vi "LogSettings.vi"(6 "ScriptName":string, 7 "Operation":T2, 8 "error in (no error)":errorcluster, 11 "Log Settings":T1) -> (0 "error out":errorcluster, 3 "Settings out":T1)   [LabVIEW 2011]
uses:
  Strict Type Controls/Settings Operation.ctl
  <vilib>/Utility/config.llb/Read Key (String).vi
  <vilib>/Utility/config.llb/Write Key (String).vi
  <vilib>/Utility/config.llb/NI_LVConfig.lvlib
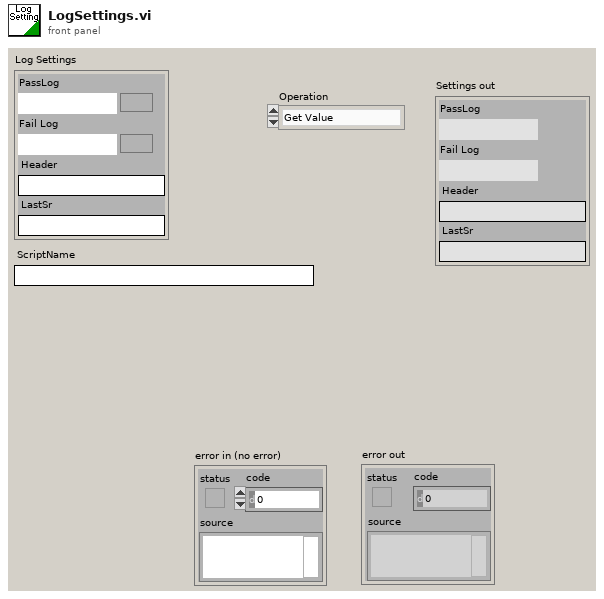
[diagram p1: front panel]
types:
  T1 = cluster{"PassLog":path, "Fail Log":path, "Header":string, "LastSr":string}
  T2 = typedef "Settings Operation.ctl" = enum8{"Get Value", "Set Value", "Read File", "Write File", "Write Stored Value"}
  T3 = typedef "NI_LVConfig.lvlib/Config Data RefNum.ctl" = refnum<k1>
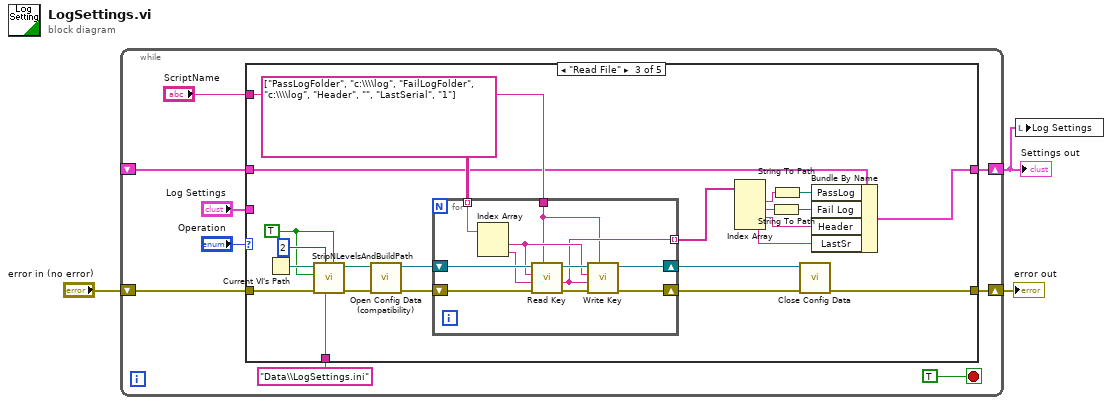
[diagram p0: block diagram]
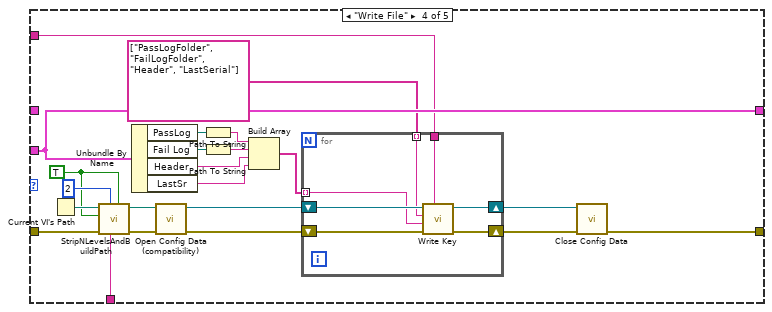
[diagram p4: hidden frame]
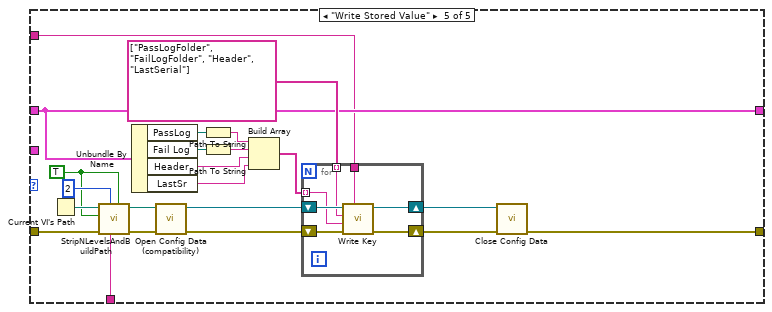
[diagram p5: hidden frame]
diagram:
  n1 = while {
    shift-right: [w11] -> w1
    shift-left: _ -> [w12]
    shift-right: [w8] -> w2
    shift-left: "error in (no error)" -> [w9]
    stop <- TRUE stop-if-true
    n2 = case shown="\"Read File\"" "Operation" {
      tunnel: w12 -> [w14 _ w27 _ w82]
      tunnel: [w14 w16 w26 w62 w82] -> w11
      tunnel: "Log Settings" -> [_ w16 _ w62 _]
      tunnel: w9 -> [w13 w15 w34 w71 w100]
      tunnel: [w13 w15 w18 w66 w95] -> w8
      tunnel: "Data\\LogSettings.ini" ("Build Path") -> [_ _ w33 w65 w94]
      tunnel: "ScriptName" -> [_ _ w28 w52 w81]
      frame "Get Value" {
      }
      frame "Set Value" {
      }
      frame "Read File" {
        w37 = TRUE ("Is File?")
        n3 = Current VI's Path() -> (path=w39:path)
        n4 = call "StripNLevelsAndBuildPath.vi"("Create Folders"=w37, "Build Path"=w33, "Strip Levels"=2, "error in(no error)"=w34, "Is File"=w37, "Path In"=w39) -> ("error out"=w35:errorcluster, "Path Out"=w36:path)  [unwired: 4 out]
        n5 = call <vilib>:"Open Config Data (compatibility).vi"("error in (no error)"=w35, "configuration file path"=w36) -> ("error out"=w32:errorcluster, "refnum"=w31:T3)  [unwired: 7 in, 1 out]
        n6 = for {
          shift-right: [w43] -> w30
          shift-left: w31 -> [w50]
          shift-right: [w45] -> w19
          shift-left: w32 -> [w49]
          tunnel: string[][] [["PassLogFolder", "c:\\\\log"], ["FailLogFolder", "c:\\\\log"], ["Header", ""], ["LastSerial", "1"]] ("appended array") -> [w48] mode=indexing
          tunnel: w28 -> [w40]
          tunnel: [w41] -> w25 mode=indexing
          n7 = Index Array(array=w48) -> (element #1=w42:string, element #2=w47:string)  [unwired: 2 in]
          n8 = call-poly <vilib>:"Read Key.vi"("section"=w40, "error in (no error)"=w49, "default value"=w47, "key"=w42, "refnum"=w50) -> ("error out"=w46:errorcluster, "value"=w41:string, "refnum out"=w44:T3)  [unwired: 1 in, 3 out]
          n9 = call-poly <vilib>:"Write Key.vi"("section"=w40, "error in (no error)"=w46, "value"=w41, "key"=w42, "refnum"=w44) -> ("error out"=w45:errorcluster, "refnum out"=w43:T3)  [unwired: 1 in, 4 out]
        }
        n10 = Index Array(array=w25) -> (element #1=w22:string, element #2=w24:string, element #3=w20:string, element #4=w17:string)  [unwired: 4 in]
        n11 = String To Path(string=w24) -> (path=w23:path)
        n12 = String To Path(string=w22) -> (path=w21:path)
        n13 = call <vilib>:"Close Config Data.vi"("error in (no error)"=w19, "refnum"=w30) -> ("error out"=w18:errorcluster)  [unwired: 1 in, 8 out]
        n14 = Bundle By Name(cluster=w27, "PassLog"=w21, "Fail Log"=w23, "Header"=w20, "LastSr"=w17) -> (w26:T1)
      }
      frame "Write File" {
        w69 = TRUE ("Is File?")
        n15 = Current VI's Path() -> (path=w72:path)
        n16 = call "StripNLevelsAndBuildPath.vi"("Create Folders"=w69, "Build Path"=w65, "Strip Levels"=2, "error in(no error)"=w71, "Is File"=w69, "Path In"=w72) -> ("error out"=w67:errorcluster, "Path Out"=w68:path)  [unwired: 4 out]
        n17 = Unbundle By Name(w62) -> ("PassLog"=w60:path, "Fail Log"=w61:path, "Header"=w55:string, "LastSr"=w51:string)
        n18 = call <vilib>:"Open Config Data (compatibility).vi"("error in (no error)"=w67, "configuration file path"=w68) -> ("error out"=w63:errorcluster, "refnum"=w64:T3)  [unwired: 7 in, 1 out]
        n19 = Path To String(path=w60) -> (string=w56:string)
        n20 = Path To String(path=w61) -> (string=w57:string)
        n21 = Build Array(w56, w57, w55, w51) -> (w54:string[])
        n22 = for {
          tunnel: w54 -> [w75] mode=indexing
          shift-right: [w77] -> w59
          shift-left: w64 -> [w79]
          shift-right: [w76] -> w58
          shift-left: w63 -> [w78]
          tunnel: string[] ["PassLogFolder", "FailLogFolder", "Header", "LastSerial"] ("appended array") -> [w74] mode=indexing
          tunnel: w52 -> [w73]
          n23 = call-poly <vilib>:"Write Key.vi"("section"=w73, "error in (no error)"=w78, "value"=w75, "key"=w74, "refnum"=w79) -> ("error out"=w76:errorcluster, "refnum out"=w77:T3)  [unwired: 1 in, 4 out]
        }
        n24 = call <vilib>:"Close Config Data.vi"("error in (no error)"=w58, "refnum"=w59) -> ("error out"=w66:errorcluster)  [unwired: 1 in, 8 out]
      }
      frame "Write Stored Value" {
        w98 = TRUE ("Is File?")
        n25 = Current VI's Path() -> (path=w101:path)
        n26 = call "StripNLevelsAndBuildPath.vi"("Create Folders"=w98, "Build Path"=w94, "Strip Levels"=2, "error in(no error)"=w100, "Is File"=w98, "Path In"=w101) -> ("error out"=w96:errorcluster, "Path Out"=w97:path)  [unwired: 4 out]
        n27 = Unbundle By Name(w82) -> ("PassLog"=w90:path, "Fail Log"=w91:path, "Header"=w85:string, "LastSr"=w80:string)
        n28 = call <vilib>:"Open Config Data (compatibility).vi"("error in (no error)"=w96, "configuration file path"=w97) -> ("error out"=w92:errorcluster, "refnum"=w93:T3)  [unwired: 7 in, 1 out]
        n29 = Path To String(path=w90) -> (string=w86:string)
        n30 = Path To String(path=w91) -> (string=w87:string)
        n31 = Build Array(w86, w87, w85, w80) -> (w84:string[])
        n32 = for {
          tunnel: w84 -> [w104] mode=indexing
          shift-right: [w106] -> w89
          shift-left: w93 -> [w108]
          shift-right: [w105] -> w88
          shift-left: w92 -> [w107]
          tunnel: string[] ["PassLogFolder", "FailLogFolder", "Header", "LastSerial"] ("appended array") -> [w103] mode=indexing
          tunnel: w81 -> [w102]
          n33 = call-poly <vilib>:"Write Key.vi"("section"=w102, "error in (no error)"=w107, "value"=w104, "key"=w103, "refnum"=w108) -> ("error out"=w105:errorcluster, "refnum out"=w106:T3)  [unwired: 1 in, 4 out]
        }
        n34 = call <vilib>:"Close Config Data.vi"("error in (no error)"=w88, "refnum"=w89) -> ("error out"=w95:errorcluster)  [unwired: 1 in, 8 out]
      }
    }
  }
  "error out" <- w2
  "Settings out" <- w1
  n35 = local write "Log Settings"(w1) -> ()
